vi "View Avis.vi"() -> ()   [LabVIEW 2022 SP3]
doc: "This example shows how to open, read, and display an AVI file in NI Vision. The VI reads the frames per second property and plays the images back at the rate specified by the AVI file."
uses:
  <vilib>/Platform/TimedLoop/XDataNode/timing_clust.ctl
  <vilib>/Platform/TimedLoop/XDataNode/nitl_modes.ctl
  <vilib>/Platform/TimedLoop/XDataNode/wakeup.ctl
  <vilib>/platform/TimedLoop/XDataNode/XDataNode.xnode
  <vilib>/Platform/TimedLoop/XDataNode/XDNodeRunTimeDep.lvlib
panel:
  out "Frame Data 2":T1
  out "Frame Data":T1
  out "Image":T2(plugin-control)
  in  "stop":bool
  out "Number of Frames 2":u32
  out "Number of Frames":u32
  out "Image 2":T2(plugin-control)
  in  "path 1":u32
  in  "path 2":u32
  in  "AVI File Path 2":path
  in  "AVI File Path":path
  # "Overview: Demonstrate the use of the AVI functions to read an AVI movie file.\nRequirements: Vision Development Software.\nInstructions: Run the VI."
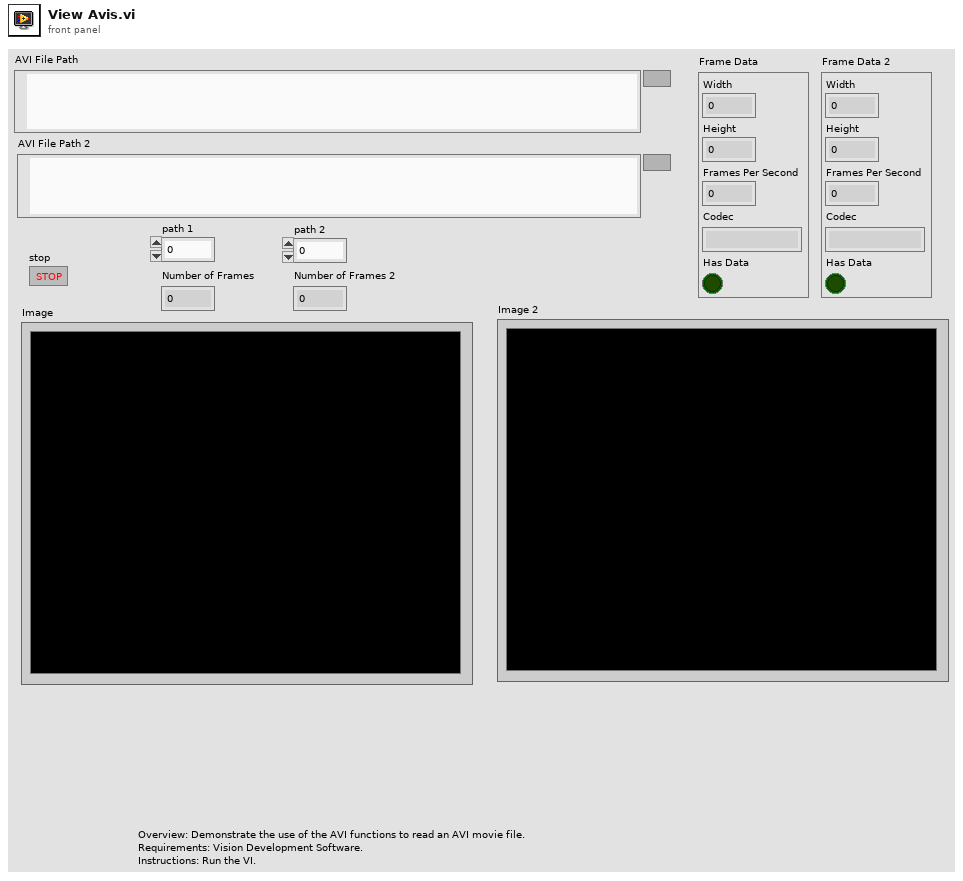
[diagram p1: front panel]
types:
  T1 = cluster{"Width":u32, "Height":u32, "Frames Per Second":u32, "Codec":string, "Has Data":bool}
  T2 = typedef "IMAQ Image.ctl" = refnum<image>
  T3 = typedef "XDNodeRunTimeDep.lvlib/timing_clust.ctl" = cluster{"Expected End [f-1]":u64, "Actual End [f-1]":u64, "Finished Late? [f-1]":bool, "Expected End [i-1]":u64, "Actual End [i-1]":u64, "Finished Late? [i-1]":bool, "Expected Start [i]":u64, "Actual Start [i]":u64, "Expected Start [f]":u64, "Actual Start [f]":u64, "Source Name":string, "Structure Name":string, "Period":i64, "Deadline":i64, "Offset":i64, "Start":i64, "Priority":i32, "Timeout":i32, "Mode":T4, "Wakeup Reason":T5, "Error":errorcluster, "Source Type":string, "Secondary Source Type":string, "Global End Time":u64, "Global Start Time":u64, "Frame Duration":u64, "Iteration Duration":u64, "Assigned CPU":i32, "I/O Scan Engine Mode":u32}
  T4 = typedef "XDNodeRunTimeDep.lvlib/nitl_modes.ctl" = enum32{"No Change", "Process missed periods, maintain original phase", "Discard missed periods, maintain original phase", "Process missed periods, ignore original phase", "Discard missed periods, ignore original phase"}
  T5 = typedef "XDNodeRunTimeDep.lvlib/wakeup.ctl" = enum32{"Normal", "Aborted", "Asynchronous wakeup", "Timing source error", "Timed loop error", "Timeout"}
  T6 = typedef "IMAQ AVI2 Refnum.ctl" = refnum<k20>
  T7 = typedef "Image Type" = u32
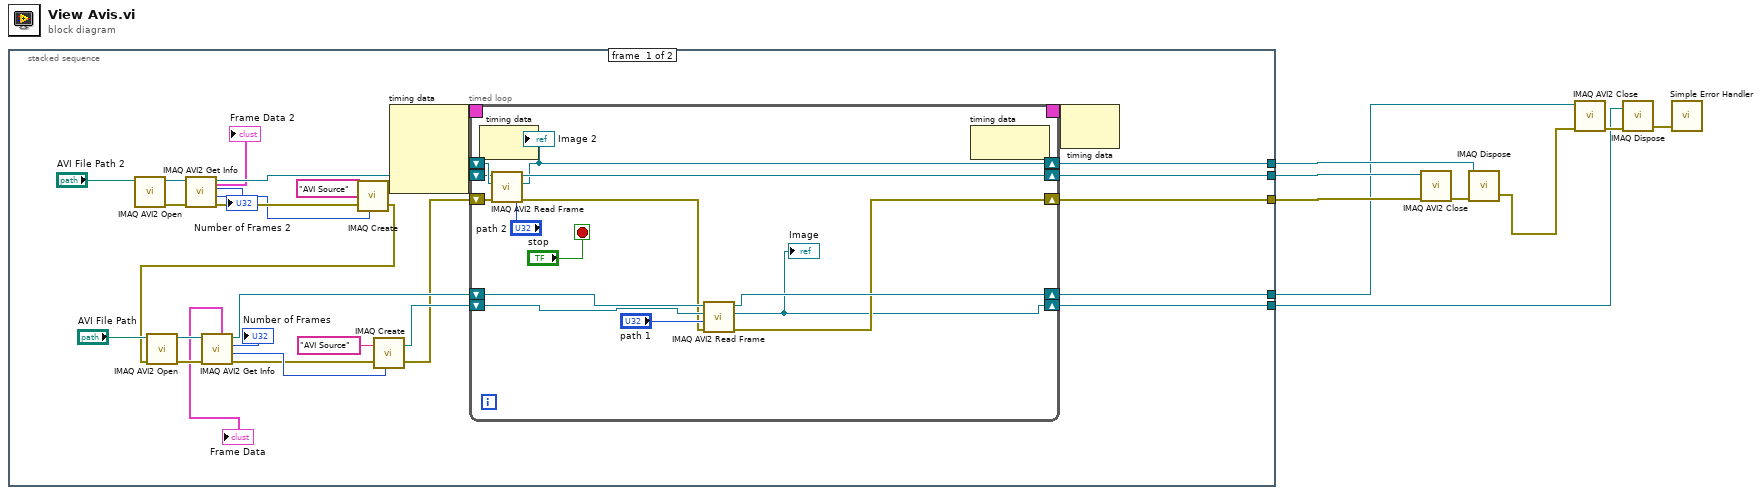
[diagram p0: block diagram]
diagram:
  n1 = stacked-sequence {
    tunnel: [w27 _] -> w9
    tunnel: [w26 _] -> w8
    tunnel: [w25 _] -> w7
    tunnel: [w13 _] -> w3
    tunnel: [w12 _] -> w1
    frame #0 {
      n2 = call "IMAQ AVI2 Open"("AVI File Path"="AVI File Path 2") -> ("error out"=w35:errorcluster, "AVI Refnum"=w34:T6)  [unwired: 2 in, 7 out]
      n3 = call "IMAQ AVI2 Get Info"("error in (no error)"=w35, "AVI Refnum"=w34) -> ("error out"=w33:errorcluster, "Image Type"=w30:T7, "Number of Frames"=→"Number of Frames 2":u32, "AVI Refnum (duplicate)"=w31:T6, "Frame Data"=→"Frame Data 2":T1)  [unwired: 5 out]
      n4 = call "IMAQ Create"("Image Name"="AVI Source", "Image Type"=w30, "error in (no error)"=w33) -> ("New Image"=w32:T2, "error out"=w15:errorcluster)  [unwired: 1 in, 1 out]
      n5 = call "IMAQ AVI2 Open"("error in (no error)"=w15, "AVI File Path"="AVI File Path") -> ("error out"=w19:errorcluster, "AVI Refnum"=w20:T6)  [unwired: 1 in, 7 out]
      n6 = call "IMAQ AVI2 Get Info"("error in (no error)"=w19, "AVI Refnum"=w20) -> ("error out"=w21:errorcluster, "Image Type"=w22:T7, "Number of Frames"=→"Number of Frames":u32, "AVI Refnum (duplicate)"=w16:T6, "Frame Data"=→"Frame Data":T1)  [unwired: 5 out]
      n7 = call "IMAQ Create"("Image Name"="AVI Source", "Image Type"=w22, "error in (no error)"=w21) -> ("New Image"=w17:T2, "error out"=w14:errorcluster)  [unwired: 1 in, 1 out]
      n8 = node-c288() -> (w38:T3)  [unwired: 4 in]
      n9 = timed-loop {
        shift-right: [w49] -> w26
        shift-left: w32 -> [w51]
        shift-right: [w52] -> w25
        shift-left: w31 -> [w50]
        shift-right: [w40] -> w27
        shift-left: w14 -> [w48]
        timing: w38 -> [_]
        timing-out: [_] -> w37
        shift-right: [w39] -> w12
        shift-left: w17 -> [w43]
        shift-right: [w42] -> w13
        shift-left: w16 -> [w44]
        stop <- "stop" stop-if-true
        n10 = node-c288() -> ()  [unwired: 1 in, 1 out]
        n11 = call "IMAQ AVI2 Read Frame"("error in (no error)"=w48, "Frame Number"="path 2", "Image"=w51, "AVI Refnum"=w50) -> ("error out"=w41:errorcluster, "Image Out"=w49:T2, "AVI Refnum (duplicate)"=w52:T6)  [unwired: 5 out]
        "Image 2" <- w49
        n12 = call "IMAQ AVI2 Read Frame"("error in (no error)"=w41, "Frame Number"="path 1", "Image"=w43, "AVI Refnum"=w44) -> ("error out"=w40:errorcluster, "Image Out"=w39:T2, "AVI Refnum (duplicate)"=w42:T6)  [unwired: 5 out]
        "Image" <- w39
        n13 = node-c288() -> ()  [unwired: 1 in, 1 out]
      }
      n14 = node-c288(w37) -> ()  [unwired: 1 out]
    }
    frame #1 {
    }
  }
  n15 = call "IMAQ AVI2 Close"("error in (no error)"=w9, "AVI Refnum"=w7) -> ("error out"=w4:errorcluster)  [unwired: 9 out]
  n16 = call "IMAQ Dispose"("Image"=w8, "error in (no error)"=w4) -> ("error out"=w2:errorcluster)  [unwired: 1 in, 3 out]
  n17 = call "IMAQ AVI2 Close"("error in (no error)"=w2, "AVI Refnum"=w3) -> ("error out"=w6:errorcluster)  [unwired: 9 out]
  n18 = call "IMAQ Dispose"("Image"=w1, "error in (no error)"=w6) -> ("error out"=w5:errorcluster)  [unwired: 1 in, 3 out]
  n19 = call <vilib>:"Simple Error Handler.vi"("error in (no error)"=w5) -> ()  [unwired: 1 in, 8 out]
